vi "ProcessAOUpdates.vi"(11 "MockAccelSettings":T1={"BufferUpdateFIFO"="MockAccelCommand", "VoltageMemory"="MockAccelerometerMemory"}) -> ()   [LabVIEW 2016, in "FPGAMockAccel.lvlib"]
uses:
  FPGAMockAccel.lvlib
  DataTypes/MockAccelSettings.ctl
  <vilib>/rvi/Emulation/niFpgaGetClockAttributes.vi
  <vilib>/rvi/Emulation/niFpgaSctlEmulationGetInTimedLoop.vi
  <vilib>/rvi/Emulation/niFpgaEmulationReportErrorSimple.vi
  <vilib>/rvi/Emulation/niFpgaCriticalErrorInLSC.vi
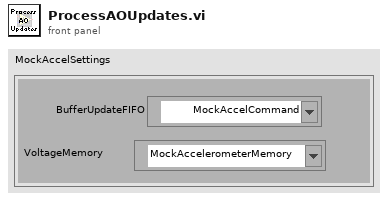
[diagram p1: front panel]
types:
  T1 = typedef "FPGAMockAccel.lvlib/MockAccelSettings.ctl" = cluster{"BufferUpdateFIFO":refnum<k21>, "VoltageMemory":refnum<k21>}
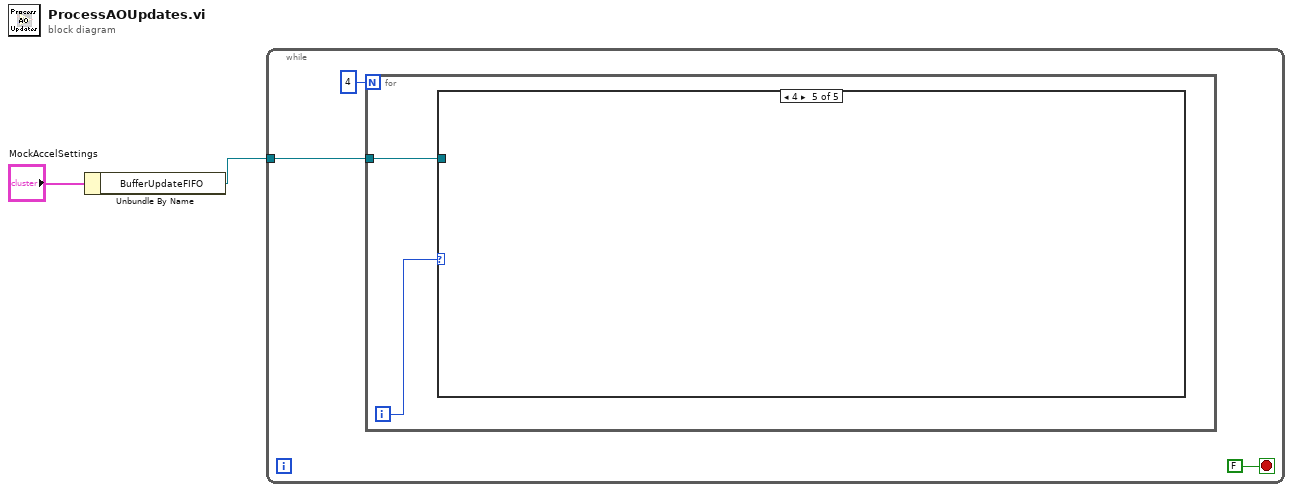
[diagram p0: block diagram]
diagram:
  n1 = Unbundle By Name("MockAccelSettings") -> ("BufferUpdateFIFO"=w1:refnum<k21>)
  n2 = while {
    tunnel: w1 -> [w4]
    stop <- FALSE stop-if-true
    n3 = for {
      N: 4 -> [_]
      tunnel: w4 -> [w7]
      i -> [w6]
      n4 = case shown="4" w6 {
        tunnel: w7 -> [_ _ _ _ _]
        frame 0, Default {
        }
        frame 1 {
        }
        frame 2 {
        }
        frame 3 {
        }
        frame 4 {
        }
      }
    }
  }
